vi "merFISH_define_DAPI_parameters.vi"(5 "Probe Refnum":refnum<vi>, 6 "Probe Names":string[][](array[string])=[["DAPI", "0"]], 7 "Laser Refnum":refnum<vi>, 8 "error in":errorcluster, 9 "Photobleaching Refnum":refnum<vi>, 10 "Hybridization Refnum":refnum<vi>, 11 "Laser lines array  IN":dbl[][](array[numeric])) -> (0 "error out":errorcluster)   [LabVIEW 2015]
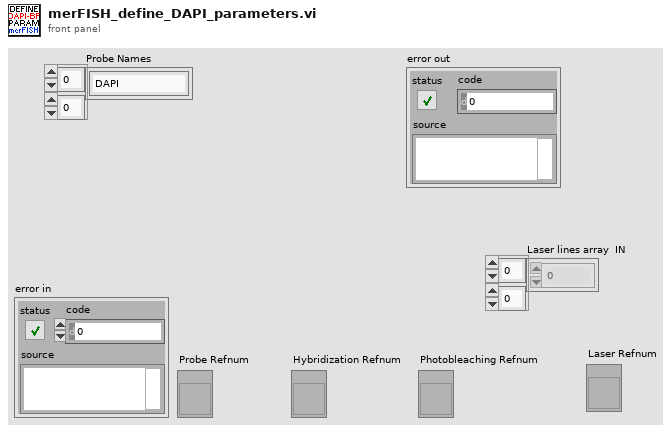
[diagram p1: front panel]
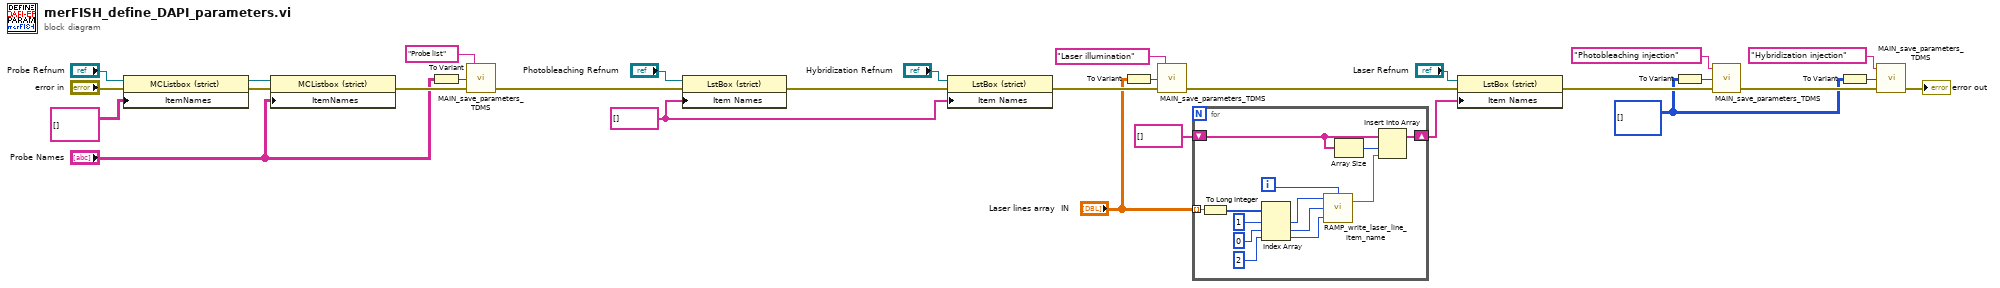
[diagram p0: block diagram]
diagram:
  w1 = i32[][] [] ("Hybridization procedure")
  w23 = string[] [] ("Item Names")
  n1 = property class="MCListbox (strict)"(reference="Probe Refnum", error in="error in", "ItemNames"=string[][] [] ("Item Names")) -> (reference out=w27:refnum<vi>, error out=w26:errorcluster)
  n2 = property class="MCListbox (strict)"(reference=w27, error in=w26, "ItemNames"="Probe Names") -> (error out=w16:errorcluster)  [unwired: 1 out]
  n3 = To Variant(anything="Probe Names") -> (Variant=w17:variant)
  n4 = call "MAIN_save_parameters_TDMS.vi"("error in"=w16, "Data"=w17, "Channel name"="Probe list" ("group name")) -> ("error out"=w14:errorcluster)  [unwired: 2 in]
  n5 = property class="LstBox (strict)"(reference="Photobleaching Refnum", error in=w14, "Item Names"=w23) -> (error out=w24:errorcluster)  [unwired: 1 out]
  n6 = property class="LstBox (strict)"(reference="Hybridization Refnum", error in=w24, "Item Names"=w23) -> (error out=w11:errorcluster)  [unwired: 1 out]
  n7 = To Variant(anything="Laser lines array  IN") -> (Variant=w12:variant)
  n8 = call "MAIN_save_parameters_TDMS.vi"("error in"=w11, "Data"=w12, "Channel name"="Laser illumination" ("group name")) -> ("error out"=w10:errorcluster)  [unwired: 2 in]
  n9 = for {
    tunnel: "Laser lines array  IN" -> [w43] mode=indexing
    shift-right: [w31] -> w20
    shift-left: string[] [] ("appended array") -> [w33]
    i -> [w35]
    n10 = To Long Integer(number=w43) -> (32bit integer=w36:i32[])
    n11 = Index Array(array=w36, index #1=1 ("index"), index #2=0 ("index"), index #3=2 ("index")) -> (element #1=w37:i32, element #2=w39:i32, element #3=w38:i32)
    n12 = call "RAMP_write_laser_line_item_name.vi"("Laser line number"=w35, "Laser application"=w38, "Power or time"=w39, "Laser line"=w37) -> ("Item name"=w34:string)  [unwired: 1 in]
    n13 = Array Size(array=w33) -> (size(s)=w32:i32)
    n14 = Insert Into Array(array=w33, index=w32, new element=w34) -> (w31:string[])
  }
  n15 = property class="LstBox (strict)"(reference="Laser Refnum", error in=w10, "Item Names"=w20) -> (error out=w3:errorcluster)  [unwired: 1 out]
  n16 = To Variant(anything=w1) -> (Variant=w4:variant)
  n17 = call "MAIN_save_parameters_TDMS.vi"("error in"=w3, "Data"=w4, "Channel name"="Photobleaching injection" ("group name")) -> ("error out"=w8:errorcluster)  [unwired: 2 in]
  n18 = To Variant(anything=w1) -> (Variant=w7:variant)
  n19 = call "MAIN_save_parameters_TDMS.vi"("error in"=w8, "Data"=w7, "Channel name"="Hybridization injection" ("group name")) -> ("error out"=→"error out":errorcluster)  [unwired: 2 in]
